vi "QE Read.vi"(8 "Error In":errorcluster={"status"=TRUE, "code"=5001, "source"="LVH-LINX.lvlib:Generate Error.vi<ERR>\nA timeout occured while waiting for the LINX device to respond."}, 10 "QE Channels":u8[](array[numeric])=[0], 11 "LINX Device Config 2":T1={"Interface"=enum."Serial", "COM Port"="COM5", "TCP Configuration"={"IP Address"="", "Port"=0}, "Device Family"=0, "Device ID"=0, "Device Name"="", "TCP Ref"=refnum, "Channels"={"DI Channels"=[], "DO Channels"=[], "AI"=[], "AO"=[], "PWM"=[], "QE"=[], "UART"=[], "I2C 2"=[], "SPI"=[], "CAN"=[], "AI Ref (V)"=0.0, "AO Resolution (Bits)"=0, "AO Ref (V)"=0.0}}) -> (0 "Error Out":errorcluster={"status"=TRUE, "code"=5001, "source"="LVH-LINX.lvlib:Generate Error.vi<ERR>\nA timeout occured while waiting for the LINX device to respond."}, 2 "Counters":i32[](array[numeric]), 3 "LINX Device Config":T1={"Interface"=enum."Serial", "COM Port"="COM5", "TCP Configuration"={"IP Address"="", "Port"=0}, "Device Family"=0, "Device ID"=0, "Device Name"="", "TCP Ref"=refnum, "Channels"={"DI Channels"=[], "DO Channels"=[], "AI"=[], "AO"=[], "PWM"=[], "QE"=[], "UART"=[], "I2C 2"=[], "SPI"=[], "CAN"=[], "AI Ref (V)"=0.0, "AO Resolution (Bits)"=0, "AO Ref (V)"=0.0}})   [LabVIEW 2013, in "LVH-LINX.lvlib" / "Device.lvlib"]
uses:
  Device.lvlib
  Type Defs/LINX Device Config.ctl
  Type Defs/Interface.ctl
  Type Defs/TCP Config.ctl
  Type Defs/Channels.ctl
  Type Defs/Error Type.ctl
  LVH-LINX.lvlib
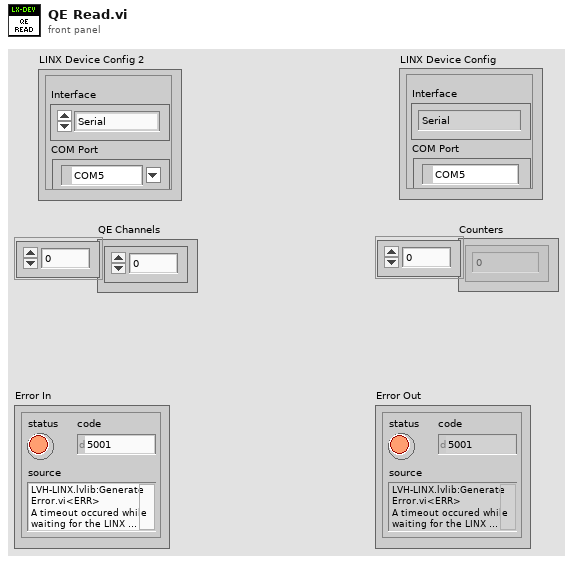
[diagram p1: front panel]
types:
  T1 = typedef "LVH-LINX.lvlib/Device.lvlib/LINX Device Config.ctl" = cluster{"Interface":T2, "COM Port":refnum<visa-resource-name>, "TCP Configuration":T3, "Device Family":u8, "Device ID":u8, "Device Name":string, "TCP Ref":refnum<k5>, "Channels":T4}
  T2 = typedef "LVH-LINX.lvlib/Interface.ctl" = enum16{"Serial", "TCP"}
  T3 = typedef "LVH-LINX.lvlib/Device.lvlib/TCP Config.ctl" = cluster{"IP Address":string, "Port":u16}
  T4 = typedef "LVH-LINX.lvlib/Channels.ctl" = cluster{"DI Channels":u8[], "DO Channels":u8[], "AI":u8[], "AO":u8[], "PWM":u8[], "QE":u8[], "UART":u8[], "I2C 2":u8[], "SPI":u8[], "CAN":u8[], "AI Ref (V)":dbl, "AO Resolution (Bits)":u8, "AO Ref (V)":dbl}
  T5 = typedef "LVH-LINX.lvlib/Error Type.ctl" = enum16{"Unknown", "Timeout", "Corrupt Return Packet", "Unable To Connect", "Command Not Supported", "Channel DNE", "Invalid COM Config", "Firmware Version Mismatch", "myRIO Support"}
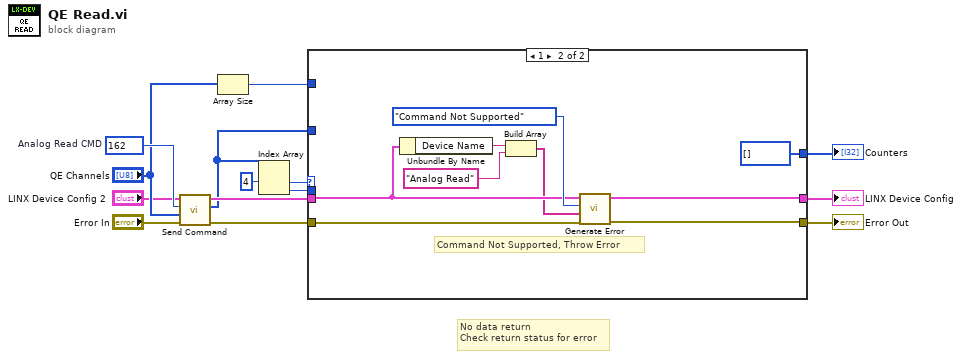
[diagram p0: block diagram]
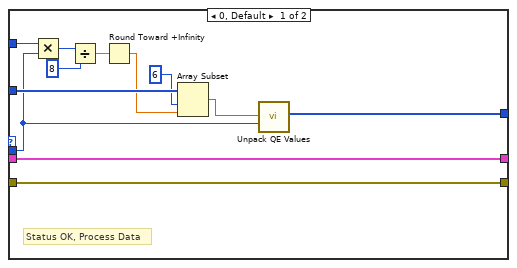
[diagram p2: hidden frame]
diagram:
  w13 = u16 162  # Analog Read CMD
  # "No data return\nCheck return status for error"
  n1 = call "Send Command.vi"("Error In"="Error In", "ARGS"="QE Channels", "CMD"=w13, "LINX Device Config"="LINX Device Config 2") -> ("Error Out"=w7:errorcluster, "Response"=w6:u8[], "LINX Device Config"=w9:T1)  [unwired: 4 in, 1 out]
  n2 = Array Size(array="QE Channels") -> (size(s)=w4:i32)
  n3 = Index Array(array=w6, index #1=4 ("index")) -> (element #1=w11:u8, element #2=w3:u8)  [unwired: 1 in]
  n4 = case shown="1" w11 {
    tunnel: [w19 w33] -> w10
    tunnel: w9 -> [w19 w29]
    tunnel: [w18 w34] -> w8
    tunnel: w7 -> [w18 w35]
    tunnel: w6 -> [w26 _]
    tunnel: w4 -> [w25 _]
    tunnel: w3 -> [w16 _]
    tunnel: [w15 i32[] [] ("QE Counts")] -> w1
    frame 0, Default {
      # "Status OK, Process Data"
      n5 = Multiply(x=w25, y=w16) -> (x*y=w24:i32)
      n6 = Divide(x=w24, y=8) -> (x/y=w22:dbl)
      n7 = Round Toward +Infinity(x=w22) -> (ceil(x): smallest int >= x=w20:dbl)
      n8 = Array Subset(array=w26, index=6, length=w20) -> (w17:u8[])
      n9 = call "Unpack QE Values.vi"("Resolution"=w16, "Values"=w17) -> ("QE Counts"=w15:i32[])  [unwired: 9 in]
    }
    frame 1 {
      # "Command Not Supported, Throw Error"
      n10 = Unbundle By Name(w29) -> ("Device Name"=w31:string)
      n11 = Build Array(w31, "Analog Read") -> (w28:string[])
      n12 = call "Generate Error.vi"("Error In"=w35, "Arguments"=w28, "Error Type"=Error_Type."Command Not Supported", "LINX Device Config"=w29) -> ("Error Out"=w34:errorcluster, "LINX Device Config"=w33:T1)  [unwired: 6 in]
    }
  }
  "Error Out" <- w8
  "LINX Device Config" <- w10
  "Counters" <- w1
